vi "divide.vi"() -> ()   [LabVIEW 2020]
panel:
  out "ERROR":bool
  out "RESULT":dbl
  in  "divisor":dbl
  out "random_number":dbl
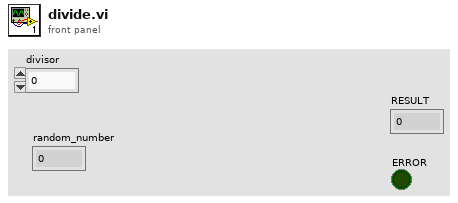
[diagram p1: front panel]
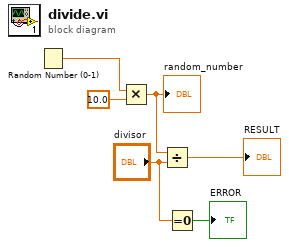
[diagram p0: block diagram]
diagram:
  n1 = Random Number (0-1)() -> (number: 0 to 1=w5:dbl)
  n2 = Multiply(x=w5, y=10.0) -> (x*y=w4:dbl)
  "random_number" <- w4
  n3 = Divide(x=w4, y="divisor") -> (x/y=→"RESULT":dbl)
  n4 = Equal To 0?(x="divisor") -> (x = 0?=→"ERROR":bool)
